vi "Test_freq_generator_5772.vi"() -> ()   [LabVIEW 2013]
uses:
  <vilib>/measure/maspectr.llb/Power Spectrum and PSD Export Mode.ctl
  <vilib>/measure/maspectr.llb/FFT Power Spectrum and PSD for 1 Chan (CDB).vi
  <vilib>/measure/NI_MAPro.lvlib
panel:
  out "power spectrum":cluster{"f0":dbl, "df":dbl, "magnitude":dbl[]}(graph)
  out "Cos":fxp<+/-,16,0>[][](array[numeric])
  out "simdata":i16[][](array[numeric])
  out "Sin":fxp<+/-,16,0>[][](array[numeric])
  out "Waveform Graph 2":i16[](graph)
  out "Waveform Graph":dbl[][](graph)
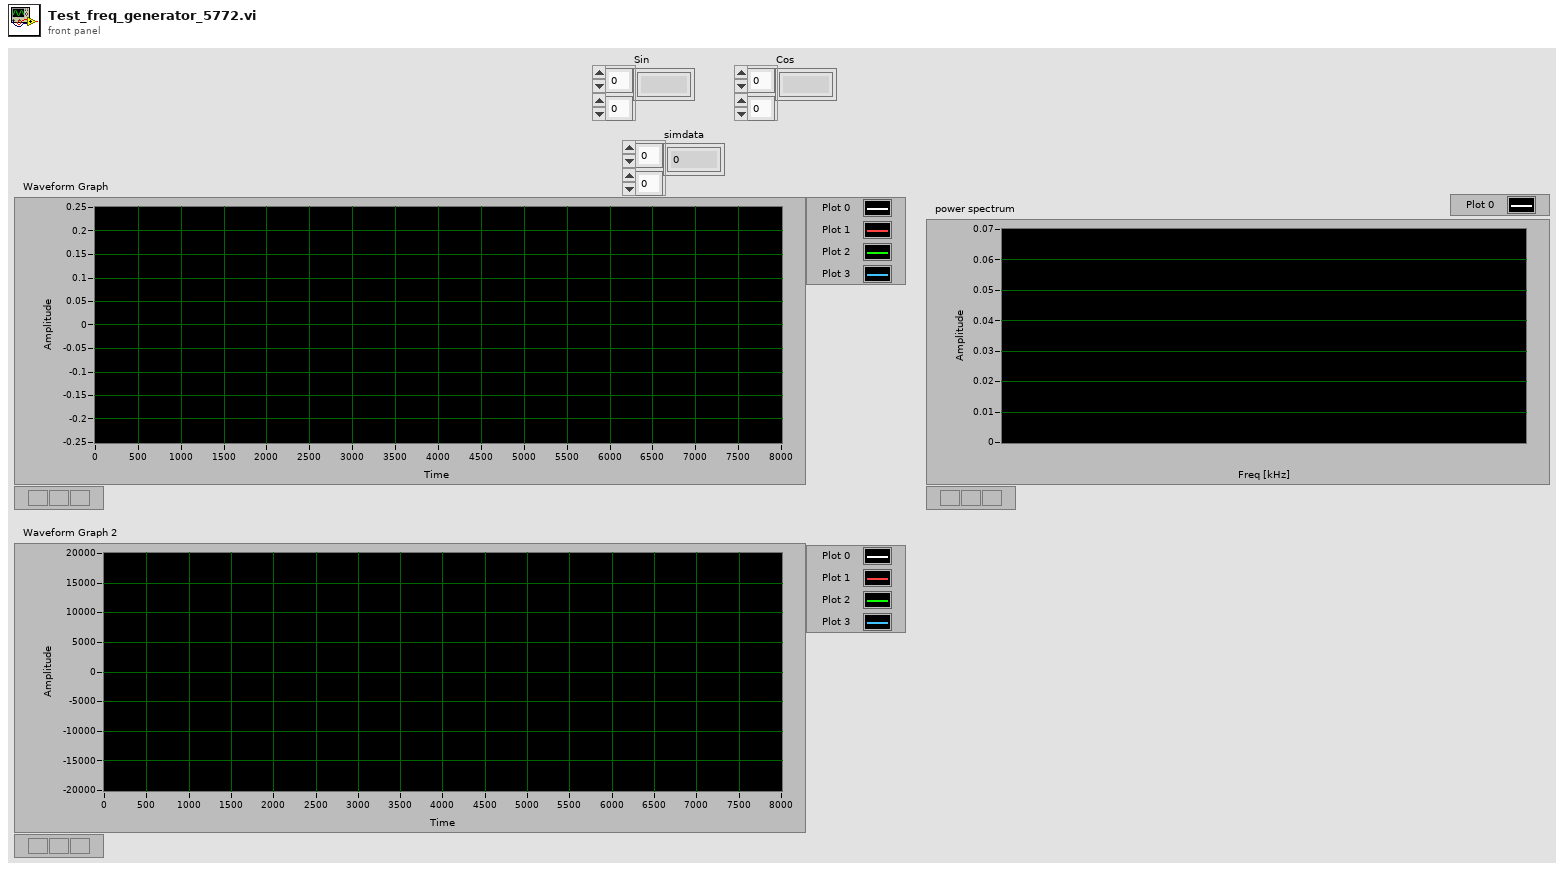
[diagram p1: front panel]
types:
  T1 = typedef "NI_MAPro.lvlib/Power Spectrum and PSD Export Mode.ctl" = u16
  T2 = typedef "I16 array size 4.ctl" = i16[]
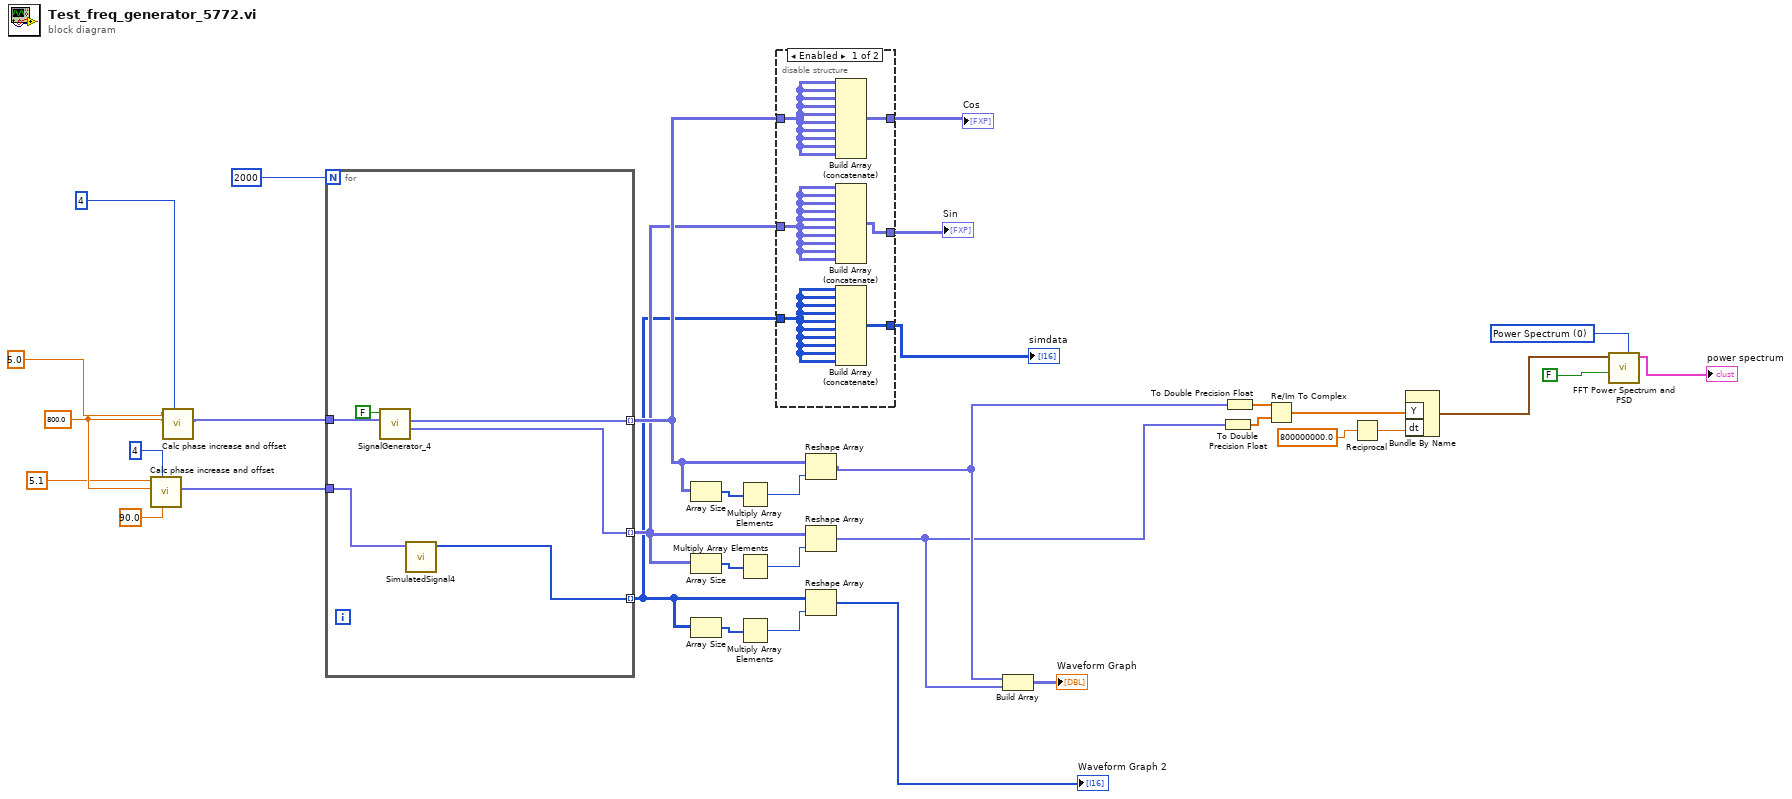
[diagram p0: block diagram]
diagram:
  w21 = T1 0 items=["Power Spectrum", "Power Spectral Density"] ("export mode")
  w33 = 800.0 ("fclk (800MHz)")
  n1 = call "Calc phase increase and offset.vi"("Phase offset (deg)"=90.0, "# of DDS"=4, "fclk (MHz)"=w33, "f_generated (MHz)"=5.1) -> ("Phase out"=w23:fxp<+,64,64>[])  [unwired: 5 in, 2 out]
  n2 = call "Calc phase increase and offset.vi"("# of DDS"=4, "fclk (MHz)"=w33, "f_generated (MHz)"=5.0) -> ("Phase out"=w24:fxp<+,64,64>[])  [unwired: 6 in, 2 out]
  n3 = for {
    N: 2000 -> [_]
    tunnel: w24 -> [w40]
    tunnel: [w39] -> w8 mode=indexing
    tunnel: w23 -> [w38]
    tunnel: [w37] -> w4 mode=indexing
    tunnel: [w35] -> w5 mode=indexing
    n4 = call "SignalGenerator_4.vi"("Phase"=w40, "reset"=FALSE) -> ("Sine out"=w35:fxp<+/-,16,0>[], "Cosine out"=w39:fxp<+/-,16,0>[])  [unwired: 8 in]
    n5 = call "SimulatedSignal4.vi"("Phase"=w38) -> ("output"=w37:T2)  [unwired: 9 in, 1 out]
  }
  n6 = Array Size(array=w8) -> (size(s)=w28:i32[])
  n7 = Array Size(array=w5) -> (size(s)=w10:i32[])
  n8 = Array Size(array=w4) -> (size(s)=w25:i32[])
  n9 = Multiply Array Elements(1:w28) -> (0:w27:i32)
  n10 = Multiply Array Elements(1:w10) -> (0:w11:i32)
  n11 = Multiply Array Elements(1:w25) -> (0:w26:i32)
  n12 = disable-structure shown="Enabled" {
    disable-tunnel: w5 -> [w46 w48]
    disable-tunnel: [w45 w49] -> w7
    disable-tunnel: [w44 w48] -> w6
    disable-tunnel: w8 -> [w43 w49]
    disable-tunnel: w4 -> [w42 w47]
    disable-tunnel: [w41 w47] -> w3
    frame Enabled {
      n13 = Build Array (concatenate)(w43, w43, w43, w43, w43, w43, w43, w43, w43, w43) -> (w45:fxp<+/-,16,0>[][])
      n14 = Build Array (concatenate)(w46, w46, w46, w46, w46, w46, w46, w46, w46, w46) -> (w44:fxp<+/-,16,0>[][])
      n15 = Build Array (concatenate)(w42, w42, w42, w42, w42, w42, w42, w42, w42, w42) -> (w41:i16[][])
    }
    frame Disabled {
    }
  }
  "Sin" <- w6
  "simdata" <- w3
  "Cos" <- w7
  n16 = Reshape Array(w8, w27) -> (w2:fxp<+/-,16,0>[])
  n17 = Reshape Array(w5, w11) -> (w1:fxp<+/-,16,0>[])
  n18 = Reshape Array(w4, w26) -> (→"Waveform Graph 2":i16[])
  n19 = Build Array(w2, w1) -> (→"Waveform Graph":fxp<+/-,16,0>[][])
  n20 = To Double Precision Float(number=w1) -> (double precision float=w14:dbl[])
  n21 = To Double Precision Float(number=w2) -> (double precision float=w15:dbl[])
  n22 = Re/Im To Complex(1:w14, 2:w15) -> (0:w13:cdb[])
  n23 = Reciprocal(x=800000000.0 ("dt")) -> (1/x=w17:dbl)
  n24 = Bundle By Name("Y"=w13, "dt"=w17) -> (w20:waveform(cdb))  [unwired: 1 in]
  n25 = call-poly <vilib>:"FFT Power Spectrum and PSD.vi"("export mode"=w21, "dB On (F)"=FALSE, "time signal"=w20) -> ("Power Spectrum / PSD"=→"power spectrum":cluster{"f0":dbl, "df":dbl, "magnitude":dbl[]})  [unwired: 5 in, 3 out]
